vi "Avviso configurazione in corso.vi"() -> ()   [LabVIEW 2019]
panel:
  out "Horizontal Graduated Bar":u8(slide) scale=0.0..100.0
  # "CONFIGURAZIONE ELETTRICA\n     DEL SISTEMA IN CORSO"
  # "ATTENDI..."
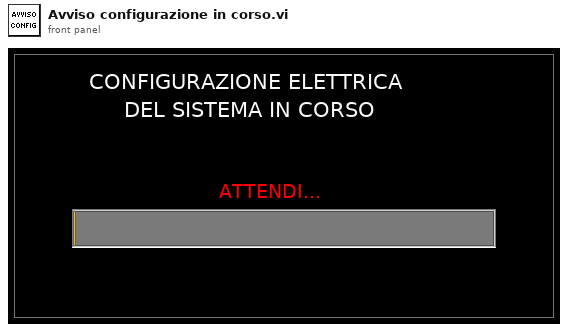
[diagram p1: front panel]
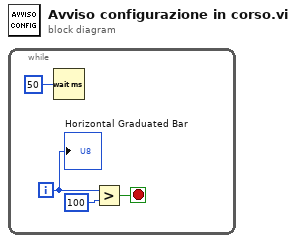
[diagram p0: block diagram]
diagram:
  n1 = while {
    i -> [w1]
    stop <- w2 stop-if-true
    n2 = Wait (ms)(milliseconds to wait=u32 50) -> ()  [unwired: 1 out]
    n3 = Greater?(x=w1, y=100) -> (0:w2:bool)
    "Horizontal Graduated Bar" <- w1
  }
